vi "Surface Force Set.vi"(8 "error in (no error)":errorcluster, 9 "Force Constants":cluster{"k0":dbl, "k1":dbl, "k2":dbl, "k3":dbl}={"k0"=1.0, "k1"=1.0, "k2"=1.0, "k3"=1.0}, 10 "Force Settings":u16(ring) items=["0", "1", "2", "3", "4"]) -> (0 "error out":errorcluster)   [LabVIEW 2021, in "Haptic Prog Interface.lvlib"]
doc: "Controls what force function the surface uses, and what constants are used in those functions.\n\n<b>Force Settings:</b>"
uses:
  Haptic Prog Interface.lvlib
  src/x64/Debug/Haptic Programming Interface.dll
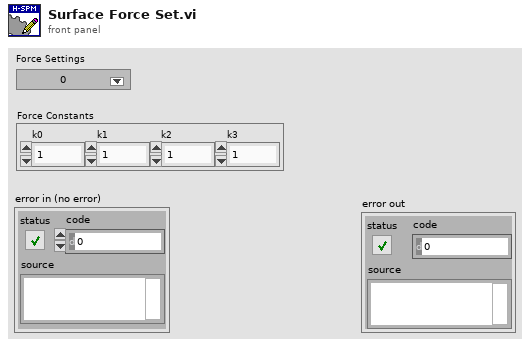
[diagram p1: front panel]
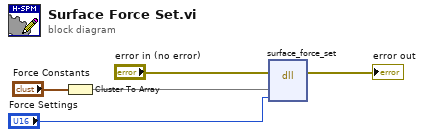
[diagram p0: block diagram]
diagram:
  n1 = Cluster To Array(cluster="Force Constants") -> (array=w3:dbl[])
  n2 = dll-call lib="C:/Users/freem/Documents/GitHub/Haptic-Programming-Interface/src/x64/Debug/Haptic Programming Interface.dll" fn="surface_force_set"(error in="error in (no error)", "input"=w3, "setting"="Force Settings") -> (error out=→"error out":errorcluster)  [unwired: 5 in, 1 out]
